vi "health.vi"() -> ()   [LabVIEW 2018]
uses:
  health_state.ctl
  health_Loop_Clust.ctl
  <vilib>/Utility/file.llb/Write To Spreadsheet File (DBL).vi
panel:
  out "Hatch Command":bool
  in  "Sample Now":bool
  out "Faults Since":string
  out "Total Faults":i16
  out "Running LED":bool
  out "Progress Bar":dbl(slide) scale=0.0..60.0
  out "Error Dialog":string="Error Message Display Box"
  out "Values":dbl[](array[numeric]) format="%.3g"
  out "Faults":bool[](array[boolean])
  out "Units":string[](array[string])
  out "Label":string[](array[string])
  out "Header":picture
  in  "Toggle Hatch":bool
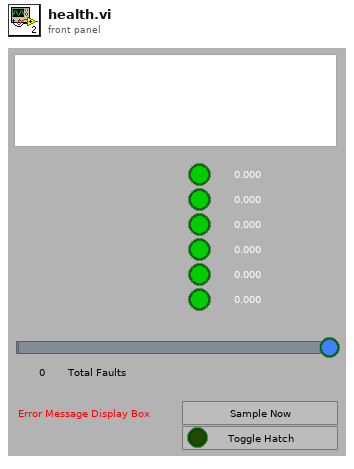
[diagram p1: front panel]
types:
  T1 = typedef "health_Loop_Clust.ctl" = cluster{"nSignals":i32, "logname":string, "time":timestamp, "dir":path, "adamSerial":cluster{"port":refnum<visa-resource-name>, "timeout":u32, "baud":u32, "dataBits":u16, "stopBits":u16, "flowControl":u16, "parity":u16, "termChar":bool, "checkSum":bool}, "fiberSerial":cluster{"port1":refnum<visa-resource-name>, "port2":refnum<visa-resource-name>, "timeout":u32, "baud":u32, "dataBits":u16, "stopBits":u16, "flowControl":u16, "parity":u16, "termChar":bool, "checkSum":bool, "fiber1On":bool, "fiber2On":bool}, "signal":cluster{"src":enum16{"adam", "fiber", "te"}[], "id":string[], "ch":string[], "descrip":string[], "units":string[], "scale":dbl[], "hi":dbl[], "lo":dbl[], "rec":bool[], "fault":bool[], "val":dbl[]}, "teSerial":cluster{"port":refnum<visa-resource-name>, "timeout":u32, "baud":u32, "dataBits":u16, "stopBits":u16, "flowControl":u16, "parity":u16, "termChar":bool, "checkSum":bool, "checkSumVal":string}, "lograte":u32, "calSwitch":bool, "logoffset":dbl}
  T2 = typedef "health_state.ctl" = enum16{"Health_Config", "Health_Wait", "Health_Read", "Health_Log", "Health_Exit"}
  T3 = typedef "imagedata.ctl" = cluster{"image type":i32, "image depth":i32, "image":u8[], "mask":u8[], "colors":u32[], "Rectangle":cluster{"left":i16, "top":i16, "right":i16, "bottom":i16}}
  T4 = cluster{"port":refnum<visa-resource-name>, "timeout":u32, "baud":u32, "dataBits":u16, "stopBits":u16, "flowControl":u16, "parity":u16, "termChar":bool, "checkSum":bool}
  T5 = typedef "LVPointTypeDef.ctl" = cluster{"Horizontal":i16, "Vertical":i16}
  T6 = typedef "LVRectTypeDef.ctl" = cluster{"Left":i16, "Top":i16, "Right":i16, "Bottom":i16}
  T7 = cluster{"port1":refnum<visa-resource-name>, "port2":refnum<visa-resource-name>, "timeout":u32, "baud":u32, "dataBits":u16, "stopBits":u16, "flowControl":u16, "parity":u16, "termChar":bool, "checkSum":bool, "fiber1On":bool, "fiber2On":bool}
  T8 = cluster{"port":refnum<visa-resource-name>, "timeout":u32, "baud":u32, "dataBits":u16, "stopBits":u16, "flowControl":u16, "parity":u16, "termChar":bool, "checkSum":bool, "checkSumVal":string}
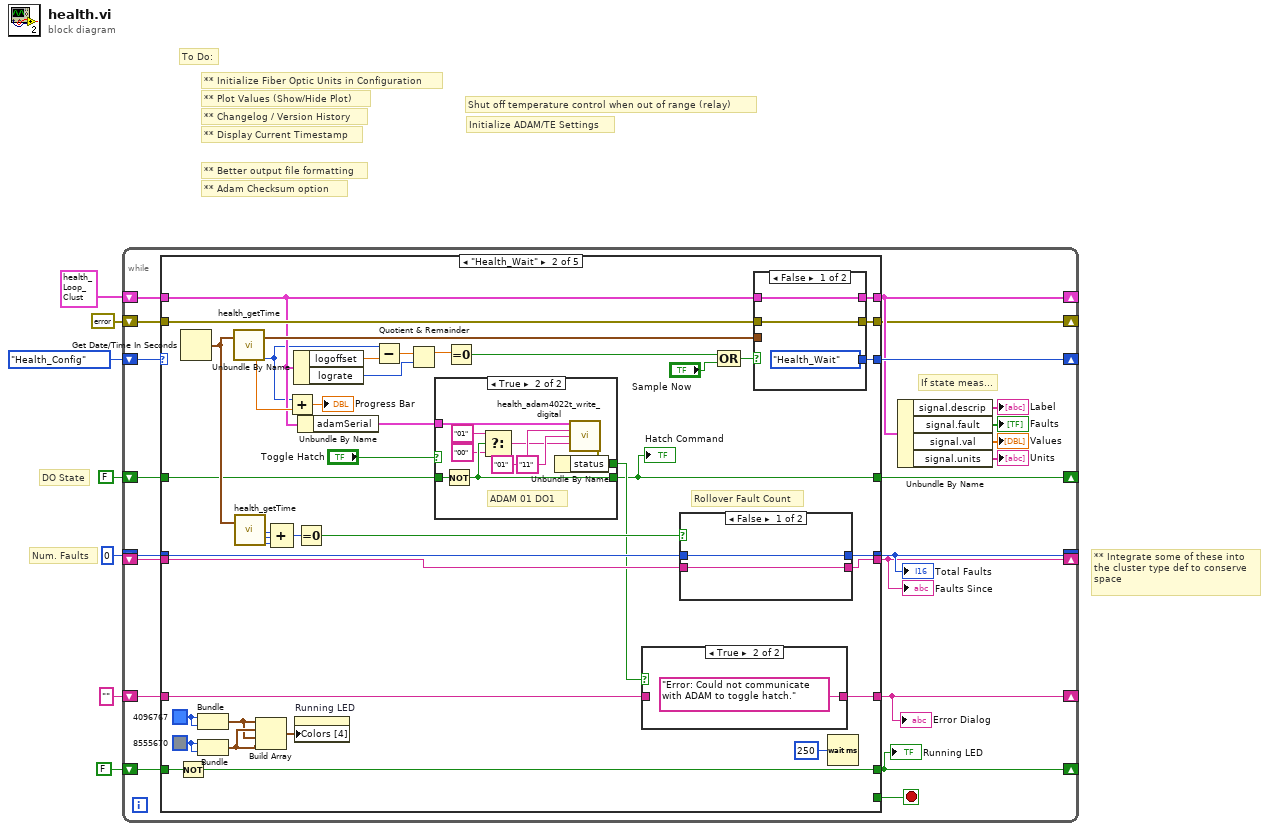
[diagram p0: block diagram]
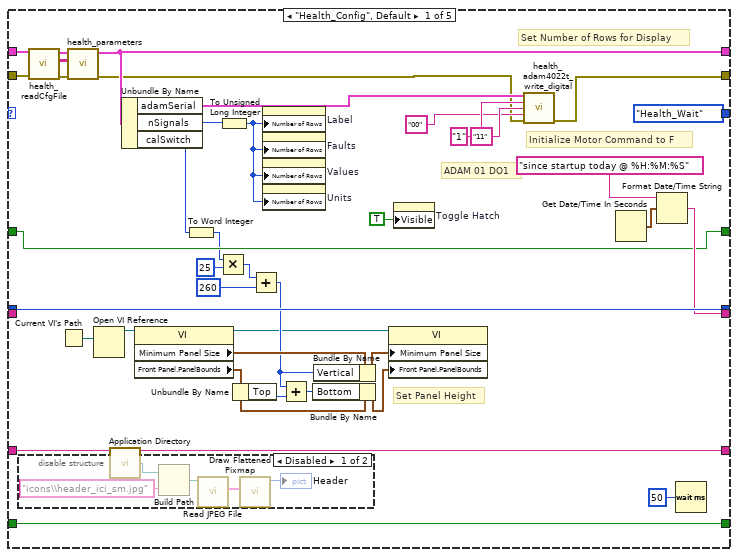
[diagram p2: hidden frame]
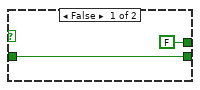
[diagram p5: hidden frame]
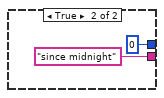
[diagram p6: hidden frame]
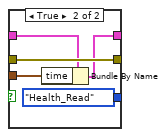
[diagram p7: hidden frame]
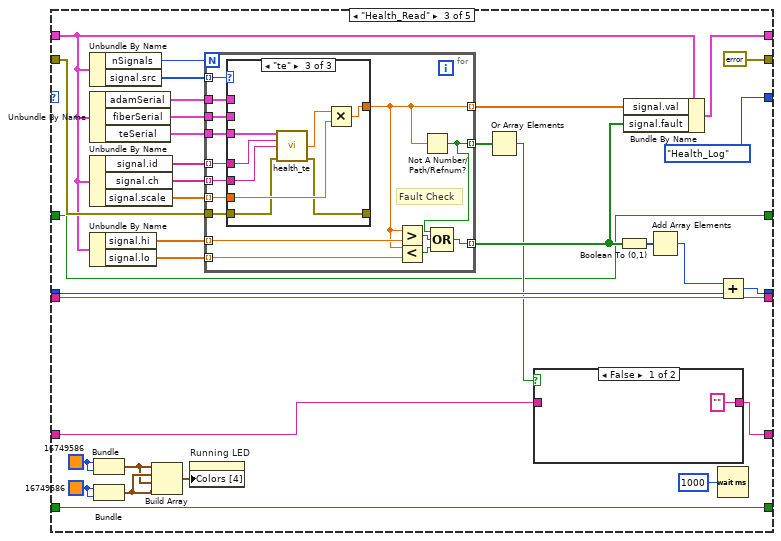
[diagram p8: hidden frame]
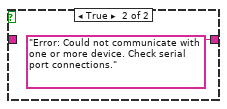
[diagram p9: hidden frame]
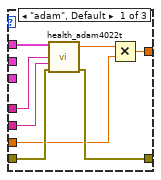
[diagram p10: hidden frame]
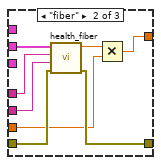
[diagram p11: hidden frame]
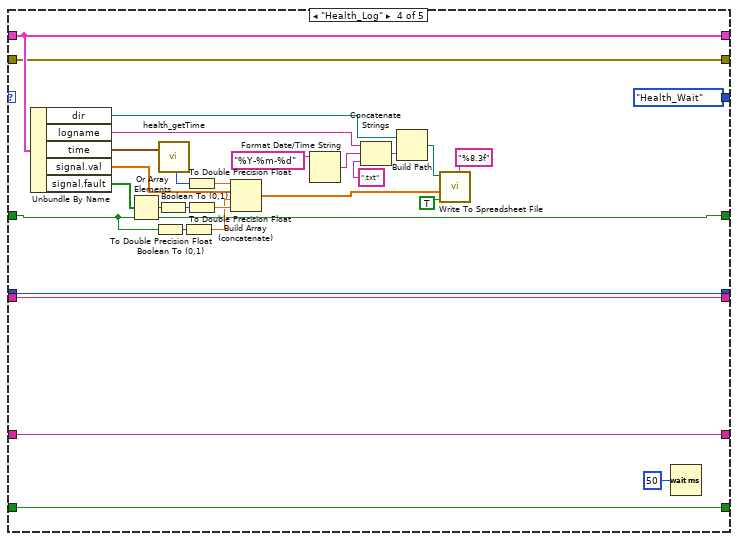
[diagram p12: hidden frame]
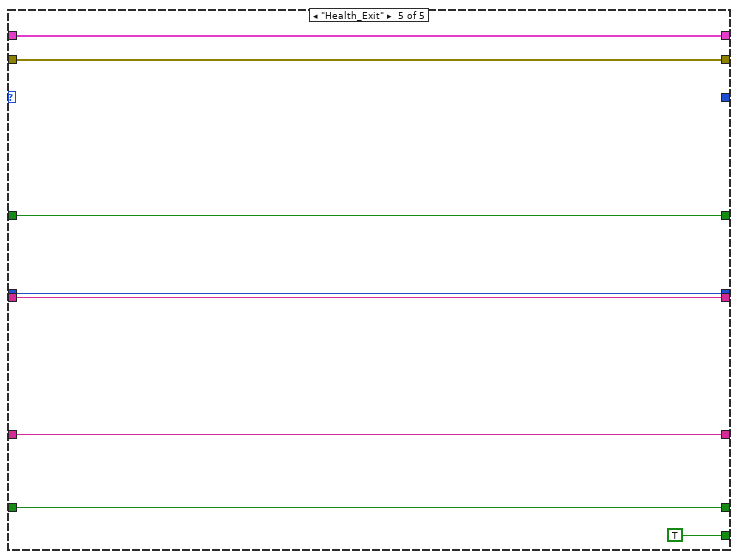
[diagram p13: hidden frame]
diagram:
  # "DO State"
  # "Initialize ADAM/TE Settings"
  # "Shut off temperature control when out of range (relay)"
  # "** Integrate some of these into\nthe cluster type def to conserve\nspace"
  # "** Changelog / Version History"
  # "** Plot Values (Show/Hide Plot)"
  # "** Display Current Timestamp"
  # "** Adam Checksum option"
  # "Num. Faults"
  # "** Better output file formatting"
  # "To Do:"
  # "** Initialize Fiber Optic Units in Configuration"
  n1 = while {
    shift-right: [w27] -> _
    shift-left: health_state."Health_Config" ("Enum") -> [w28]
    shift-right: [w21] -> _
    shift-left: T1 {"nSignals"=0, "logname"="", "time"=timestamp(0 s since 1904-01-01), "dir"=path "", "adamSerial"={"port"="", "timeout"=0, "baud"=0, "dataBits"=0, "stopBits"=0, "flowControl"=0, "parity"=0, "termChar"=FALSE, "checkSum"=FALSE}, "fiberSerial"={"port1"="", "port2"="", "timeout"=0, "baud"=0, "dataBits"=0, "stopBits"=0, "flowControl"=0, "parity"=0, "termChar"=FALSE, "checkSum"=FALSE, "fiber1On"=FALSE, "fiber2On"=FALSE}, "signal"={"src"=[], "id"=[], "ch"=[], "descrip"=[], "units"=[], "scale"=[], "hi"=[], "lo"=[], "rec"=[], "fault"=[], "val"=[]}, "teSerial"={"port"="", "timeout"=0, "baud"=0, "dataBits"=0, "stopBits"=0, "flowControl"=0, "parity"=0, "termChar"=FALSE, "checkSum"=FALSE, "checkSumVal"=""}, "lograte"=0, "calSwitch"=FALSE, "logoffset"=0.0} ("hDout") -> [w26]
    shift-right: [w11] -> _
    shift-left: errorcluster {"status"=FALSE, "code"=0, "source"=""} ("Error Out") -> [w25]
    shift-right: [w23] -> _
    shift-left: FALSE -> [w24]
    shift-right: [w16] -> _
    shift-left: i16 0 -> [w17]
    shift-right: [w15] -> _
    shift-left: _ -> [w14]
    shift-right: [w13] -> _
    shift-left: "" ("Error Dialog") -> [w12]
    shift-right: [w10] -> _
    shift-left: FALSE -> [w9]
    stop <- w8 stop-if-true
    # "If state meas..."
    n2 = case shown="\"Health_Wait\"" w28 {
      tunnel: [health_state."Health_Wait" ("Enum") w110 health_state."Health_Log" ("Enum") health_state."Health_Wait" ("Enum") _] -> w27
      tunnel: w25 -> [w65 w97 w160 w216 w245]
      tunnel: [w58 w98 w161 w231 w246] -> w21
      tunnel: w26 -> [w62 w79 w145 w231 w246]
      tunnel: [w59 w106 w169 w239 w248] -> w23
      tunnel: w24 -> [w59 w107 w169 w239 w248]
      tunnel: [w56 w92 w152 w224 w243] -> w16
      tunnel: w17 -> [w56 w91 w151 w224 w243]
      tunnel: [w54 w90 w144 w218 w242] -> w15
      tunnel: w14 -> [_ w89 w144 w218 w242]
      tunnel: [w52 w77 w142 w217 w241] -> w13
      tunnel: w12 -> [w52 w76 w140 w217 w241]
      tunnel: [w29 w86 errorcluster {"status"=FALSE, "code"=0, "source"=""} ("Error Out") w216 w245] -> w11
      tunnel: [w51 w71 w137 w212 w244] -> w10
      tunnel: w9 -> [w51 w80 w137 w212 w244]
      tunnel: [_ _ _ _ TRUE ("stop")] -> w8
      frame "Health_Config", Default {
        # "Initialize Motor Command to F"
        # "ADAM 01 DO1"
        # "Set Panel Height"
        # "Set Number of Rows for Display"
        n3 = disable-structure shown="Disabled" {
          frame Disabled {
            n4 = call <vilib>:"Application Directory.vi"() -> ("Application Directory"=w67:path)
            n5 = Build Path(base path=w67, name or relative path="icons\\header_ici_sm.jpg") -> (appended path=w68:path)
            n6 = call <vilib>:"Read JPEG File.vi"("path to JPEG file"=w68) -> ("image data"=w70:T3)  [unwired: 8 in, 2 out]
            n7 = call <vilib>:"Draw Flattened Pixmap.vi"("image data"=w70) -> ("new picture"=→"Header":picture)  [unwired: 8 in]
          }
          frame Enabled {
          }
        }
        n8 = call "health_readCfgFile.vi"("error in \n(no error)"=w65) -> ("error out"=w63:errorcluster, "parameters"=w64:string[][])  [unwired: 9 in]
        n9 = Current VI's Path() -> (path=w50:path)
        n10 = call "health_parameters.vi"("error in\n(no error)"=w63, "parameters"=w64, "hDin"=w62) -> ("error out"=w30:errorcluster, "hDout"=w58:T1)  [unwired: 7 in]
        n11 = Open VI Reference(vi path=w50) -> (vi reference=w49:refnum<vi>)  [unwired: 5 in, 1 out]
        n12 = Unbundle By Name(w58) -> ("adamSerial"=w34:T4, "nSignals"=w37:i32)  [unwired: 1 out]
        n13 = property class="VI"(reference=w49) -> (reference out=w36:refnum<vi>, "Minimum Panel Size"=w41:T5, "Front Panel.PanelBounds"=w42:T6)  [unwired: 1 in, 1 out]
        n14 = To Word Integer(number=w37) -> (16bit integer=w44:i16)
        n15 = Multiply(x=w44, y=i16 25) -> (x*y=w46:i16)
        n16 = To Unsigned Long Integer(number=w37) -> (unsigned 32bit integer=w57:u32)
        n17 = Unbundle By Name(w42) -> ("Top"=w45:i16)
        n18 = Add(x=w46, y=i16 260) -> (x+y=w40:i16)
        n19 = property on="Label" class="Arr (strict)"("Number of Rows"=w57) -> ()  [unwired: 2 in, 2 out]
        n20 = property on="Faults" class="Arr (strict)"("Number of Rows"=w57) -> ()  [unwired: 2 in, 2 out]
        n21 = property on="Values" class="Arr (strict)"("Number of Rows"=w57) -> ()  [unwired: 2 in, 2 out]
        n22 = property on="Units" class="Arr (strict)"("Number of Rows"=w57) -> ()  [unwired: 2 in, 2 out]
        n23 = Add(x=w40, y=w45) -> (x+y=w43:i16)
        n24 = Bundle By Name(cluster=w42, "Bottom"=w43) -> (w38:T6)
        n25 = Bundle By Name(cluster=w41, "Vertical"=w40) -> (w39:T5)
        n26 = property class="VI"(reference=w36, "Minimum Panel Size"=w39, "Front Panel.PanelBounds"=w38) -> ()  [unwired: 1 in, 2 out]
        n27 = property on="Toggle Hatch" class="Bool"("Visible"=TRUE) -> ()  [unwired: 2 in, 2 out]
        n28 = call "health_adam4022t_write_digital.vi"(0:w34, "Address"="1", "Channel"="11", "Value"="00" ("Address"), "Error In"=w30) -> ("Error Out"=w29:errorcluster)  [unwired: 8 in, 2 out]
        n29 = Get Date/Time In Seconds() -> (seconds since 1Jan1904=w53:timestamp)
        n30 = Format Date/Time String(time format string (%c)="since startup today @ %H:%M:%S", seconds (now)=w53) -> (date/time string=w54:string)  [unwired: 1 in]
        n31 = Wait (ms)(milliseconds to wait=u32 50) -> ()  [unwired: 1 out]
      }
      frame "Health_Wait" {
        w104 = u32 8555670
        w103 = u32 4096767
        # "Rollover Fault Count"
        n32 = Not(x=w107) -> (.not. x?=w106:bool)
        n33 = Get Date/Time In Seconds() -> (seconds since 1Jan1904=w88:timestamp)
        n34 = Bundle(w103, w103) -> (w101:cluster{u32, u32})  [unwired: 1 in]
        n35 = Bundle(w104, w104) -> (w102:cluster{u32, u32})  [unwired: 1 in]
        n36 = call "health_getTime.vi"("Current Time"=w88) -> ("Fractional Seconds"=w100:dbl, "Seconds"=w74:u32)  [unwired: 11 in, 6 out]
        n37 = call "health_getTime.vi"("Current Time"=w88) -> ("Hour"=w94:u32, "Minutes"=w95:u32, "Seconds"=w96:u32)  [unwired: 11 in, 5 out]
        n38 = Build Array(w101, w102, w101, w102) -> (w105:cluster{u32, u32}[])
        n39 = Compound Arithmetic op=ADD(w94, w95, w96) -> (w108:u32)
        n40 = Add(x=w74, y=w100) -> (x+y=→"Progress Bar":dbl)
        n41 = Unbundle By Name(w79) -> ("logoffset"=w73:dbl, "lograte"=w85:u32)
        n42 = property on="Running LED" class="Bool (strict)"("Colors [4]"=w105) -> ()  [unwired: 2 in, 2 out]
        n43 = Equal To 0?(x=w108) -> (x = 0?=w93:bool)
        n44 = Unbundle By Name(w79) -> ("adamSerial"=w78:T4)
        n45 = Subtract(x=w74, y=w73) -> (x-y=w72:dbl)
        n46 = Quotient & Remainder(x=w72, y=w85) -> (x-y*floor(x/y)=w87:dbl)  [unwired: 1 out]
        n47 = case shown="True" "Toggle Hatch" {
          tunnel: [w114 w123] -> w71
          tunnel: w80 -> [w114 w124]
          tunnel: w78 -> [_ w121]
          tunnel: [FALSE ("status") w122] -> w75
          frame False {
          }
          frame True {
            # "ADAM 01 DO1"
            n48 = Not(x=w124) -> (.not. x?=w123:bool)
            n49 = Select(t="01" ("Address"), s=w123, f="00" ("Address")) -> (s? t:f=w115:string)
            n50 = call "health_adam4022t_write_digital.vi"(0:w121, "Address"="01", "Channel"="11", "Value"=w115) -> ("Error Out"=w118:errorcluster)  [unwired: 9 in, 2 out]
            n51 = Unbundle By Name(w118) -> ("status"=w122:bool)
          }
        }
        "Hatch Command" <- w71
        n52 = Equal To 0?(x=w87) -> (x = 0?=w84:bool)
        n53 = case shown="True" w75 {
          tunnel: [w111 "Error: Could not communicate with ADAM to toggle hatch." ("Error Dialog")] -> w77
          tunnel: w76 -> [w111 _]
          frame False {
          }
          frame True {
          }
        }
        n54 = case shown="False" w93 {
          tunnel: [w126 i16 0] -> w92
          tunnel: w91 -> [w126 _]
          tunnel: [w125 "since midnight" ("time format string (%c)")] -> w90
          tunnel: w89 -> [w125 _]
          frame False {
          }
          frame True {
          }
        }
        n55 = Compound Arithmetic op=OR(w84, "Sample Now") -> (w82:bool)
        n56 = case shown="False" w82 {
          tunnel: [health_state."Health_Wait" ("Enum") health_state."Health_Read" ("Enum")] -> w110
          tunnel: [w130 w132] -> w98
          tunnel: w79 -> [w130 w134]
          tunnel: [w129 w135] -> w86
          tunnel: w97 -> [w129 w135]
          tunnel: w88 -> [_ w133]
          frame False {
          }
          frame True {
            n57 = Bundle By Name(cluster=w134, "time"=w133) -> (w132:T1)
          }
        }
        n58 = Wait (ms)(milliseconds to wait=u32 250) -> ()  [unwired: 1 out]
      }
      frame "Health_Read" {
        w168 = u32 16749586
        w167 = u32 16749586
        n59 = Unbundle By Name(w145) -> ("nSignals"=w162:i32, "signal.src"=w159:enum16{"adam", "fiber", "te"}[])
        n60 = Unbundle By Name(w145) -> ("adamSerial"=w150:T4, "fiberSerial"=w149:T7, "teSerial"=w139:T8)
        n61 = Unbundle By Name(w145) -> ("signal.id"=w148:string[], "signal.ch"=w147:string[], "signal.scale"=w146:dbl[])
        n62 = Unbundle By Name(w145) -> ("signal.hi"=w158:dbl[], "signal.lo"=w157:dbl[])
        n63 = Bundle(w167, w167) -> (w165:cluster{u32, u32})  [unwired: 1 in]
        n64 = Bundle(w168, w168) -> (w166:cluster{u32, u32})  [unwired: 1 in]
        n65 = Build Array(w165, w166, w165, w166) -> (w163:cluster{u32, u32}[])
        n66 = property on="Running LED" class="Bool (strict)"("Colors [4]"=w163) -> ()  [unwired: 2 in, 2 out]
        n67 = for {
          N: w162 -> [_]
          tunnel: w148 -> [w187] mode=indexing
          tunnel: w147 -> [w186] mode=indexing
          tunnel: [w175] -> w156 mode=indexing
          tunnel: w160 -> [w179]
          tunnel: w158 -> [w185] mode=indexing
          tunnel: w157 -> [w184] mode=indexing
          tunnel: w159 -> [w183] mode=indexing
          tunnel: [w180] -> w155 mode=indexing
          tunnel: w146 -> [w178] mode=indexing
          tunnel: w150 -> [w177]
          tunnel: w149 -> [w176]
          tunnel: [w173] -> w143 mode=indexing
          tunnel: w139 -> [w174]
          # "Fault Check"
          n68 = case shown="\"te\"" w183 {
            tunnel: w187 -> [w195 w200 w208]
            tunnel: w186 -> [w194 w199 w205]
            tunnel: [w189 w201 w210] -> w175
            tunnel: w179 -> [w193 w203 w207]
            tunnel: [w192 w202 w206] -> _
            tunnel: w178 -> [w190 w196 w211]
            tunnel: w177 -> [w188 _ _]
            tunnel: w176 -> [_ w198 _]
            tunnel: w174 -> [_ _ w209]
            frame "adam", Default {
              n69 = call "health_adam4022t.vi"(0:w188, "Address"=w195, "Channel"=w194, "Error In"=w193) -> ("Value"=w191:dbl, "Error Out"=w192:errorcluster)  [unwired: 10 in]
              n70 = Multiply(x=w191, y=w190) -> (x*y=w189:dbl)
            }
            frame "fiber" {
              n71 = call "health_fiber.vi"("fiberSerial"=w198, "Address"=w200, "Channel"=w199, "Error In"=w203) -> ("Value"=w197:dbl, "Error Out"=w202:errorcluster)  [unwired: 4 in, 1 out]
              n72 = Multiply(x=w197, y=w196) -> (x*y=w201:dbl)
            }
            frame "te" {
              n73 = call "health_te.vi"("teSerial"=w209, "Hex Address"=w208, "Command"=w205, "Error In"=w207) -> ("Response"=w204:dbl, "error out"=w206:errorcluster)  [unwired: 8 in, 2 out]
              n74 = Multiply(x=w204, y=w211) -> (x*y=w210:dbl)
            }
          }
          n75 = Greater?(x=w175, y=w185) -> (0:w182:bool)
          n76 = Less?(x=w175, y=w184) -> (x < y?=w181:bool)
          n77 = Not A Number/Path/Refnum?(number/path/refnum=w175) -> (NaN/Path/Refnum?=w173:bool)
          n78 = Compound Arithmetic op=OR(w173, w182, w181) -> (w180:bool)
        }
        n79 = Or Array Elements(Boolean array=w143) -> (logical OR=w141:bool)
        n80 = case shown="False" w141 {
          tunnel: ["" ("Error Dialog") "Error: Could not communicate with one or more device. Check serial port connections." ("Error Dialog")] -> w142
          tunnel: w140 -> [_ _]
          frame False {
          }
          frame True {
          }
        }
        n81 = Boolean To (0,1)(Boolean=w155) -> (0, 1=w153:i16[])
        n82 = Bundle By Name(cluster=w145, "signal.val"=w156, "signal.fault"=w155) -> (w161:T1)
        n83 = Add Array Elements(numeric array=w153) -> (sum=w154:i16)
        n84 = Add(x=w154, y=w151) -> (x+y=w152:i16)
        n85 = Wait (ms)(milliseconds to wait=u32 1000) -> ()  [unwired: 1 out]
      }
      frame "Health_Log" {
        n86 = Unbundle By Name(w231) -> ("dir"=w229:path, "logname"=w230:string, "time"=w228:timestamp, "signal.val"=w227:dbl[], "signal.fault"=w223:bool[])
        n87 = Or Array Elements(Boolean array=w223) -> (logical OR=w222:bool)
        n88 = Boolean To (0,1)(Boolean=w212) -> (0, 1=w214:i16)
        n89 = Boolean To (0,1)(Boolean=w222) -> (0, 1=w221:i16)
        n90 = call "health_getTime.vi"("Current Time"=w228) -> ("Seconds from Midnight"=w220:u32)  [unwired: 11 in, 7 out]
        n91 = To Double Precision Float(number=w214) -> (double precision float=w213:dbl)
        n92 = To Double Precision Float(number=w220) -> (double precision float=w226:dbl)
        n93 = To Double Precision Float(number=w221) -> (double precision float=w215:dbl)
        n94 = Build Array (concatenate)(w226, w227, w213, w215) -> (w225:dbl[])
        n95 = Format Date/Time String(time format string (%c)="%Y-%m-%d") -> (date/time string=w237:string)  [unwired: 2 in]
        n96 = Concatenate Strings(w230, w237, ".txt" ("string")) -> (w238:string)
        n97 = Build Path(base path=w229, name or relative path=w238) -> (appended path=w235:path)
        n98 = call-poly <vilib>:"Write To Spreadsheet File.vi"("format (%.3f)"="%8.3f", "append to file? (new file:F)"=TRUE, "1D data"=w225, "file path (dialog if empty)"=w235) -> ()  [unwired: 4 in, 1 out]
        n99 = Wait (ms)(milliseconds to wait=u32 50) -> ()  [unwired: 1 out]
      }
      frame "Health_Exit" {
      }
    }
    "Running LED" <- w23
    "Total Faults" <- w16
    "Faults Since" <- w15
    "Error Dialog" <- w13
    n100 = Unbundle By Name(w21) -> ("signal.descrip"=→"Label":string[], "signal.fault"=→"Faults":bool[], "signal.val"=→"Values":dbl[], "signal.units"=→"Units":string[])
  }
